vi "AttrGetIsOpen.vi"(5 "LogSuspend":bool, 8 "error in":errorcluster, 11 "UdsHandleIn":T1={"LogPath"=path "", "LogEnabled"=FALSE, "isOpen"=FALSE, "LogContent"="", "Adapter"="CAN0", "MCanHandle"={"MCanAdapter"=refnum}, "TransmittId"=0, "ReceiveId"=0}) -> (0 "error out":errorcluster, 2 "State":bool, 3 "UdsHandleOut":T1={"LogPath"=path "", "LogEnabled"=FALSE, "isOpen"=FALSE, "LogContent"="", "Adapter"="CAN0", "MCanHandle"={"MCanAdapter"=refnum}, "TransmittId"=0, "ReceiveId"=0})   [LabVIEW 2011, in "Konvolucio MUDS150628.lvlib"]
uses:
  <instrlib>/Konvolucio MUDS150628/Konvolucio MUDS150628.lvlib
  <instrlib>/Konvolucio MUDS150628/Types/UdsHandleType.ctl
  <instrlib>/Konvolucio MCAN120803/Types/MCanHandleType.ctl
  C:/Program Files/National Instruments/LabVIEW 2011/instr.lib/Konvolucio MCAN120803/Private/Konvolucio.MCAN120803.dll
  Konvolucio MCAN120803/Private/Konvolucio.MCAN120803.dll
  <instrlib>/Konvolucio MCAN120803/Konvolucio MCAN120803.lvlib
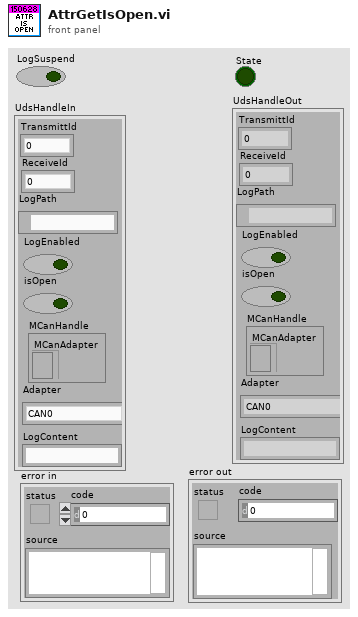
[diagram p1: front panel]
types:
  T1 = typedef "Konvolucio MUDS150628.lvlib/UdsHandleType.ctl" = cluster{"LogPath":path, "LogEnabled":bool, "isOpen":bool, "LogContent":string, "Adapter":string, "MCanHandle":T2, "TransmittId":u32, "ReceiveId":u32}
  T2 = typedef "Konvolucio MCAN120803.lvlib/MCanHandleType.ctl" = cluster{"MCanAdapter":refnum<k24>}
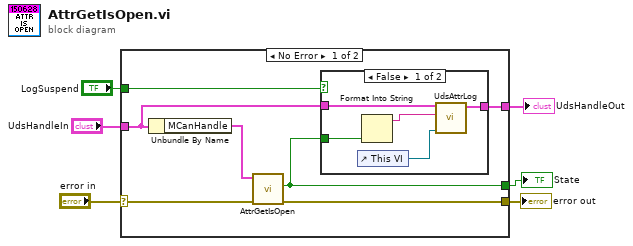
[diagram p0: block diagram]
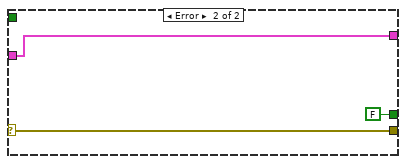
[diagram p3: hidden frame]
diagram:
  n1 = case shown="No Error" "error in" {
    selector: "error in" -> [w9 w22]
    tunnel: [w10 w22] -> w5
    tunnel: "UdsHandleIn" -> [w13 w21]
    tunnel: [w12 w21] -> w2
    tunnel: "LogSuspend" -> [w11 _]
    tunnel: [w7 FALSE ("State")] -> w6
    frame No Error {
      n2 = Unbundle By Name(w13) -> ("MCanHandle"=w8:T2)
      n3 = call <instrlib>:"AttrGetIsOpen.vi"("error in"=w9, "MCanHandleIn"=w8) -> ("error out"=w10:errorcluster, "State"=w7:bool)  [unwired: 7 in, 1 out]
      n4 = case shown="False" w11 {
        tunnel: w13 -> [w18 w19]
        tunnel: [w17 w19] -> w12
        tunnel: w7 -> [w15 _]
        frame False {
          n5 = control-ref of="This VI"() -> (w16:refnum<vi>)
          n6 = Format Into String(w15) -> (resulting string=w14:string)  [unwired: 3 in, 1 out]
          n7 = call <instrlib>:"UdsAttrLog.vi"("This VI"=w16, "Content"=w14, "UdsHandleIn"=w18) -> ("UdsHandleOut"=w17:T1)  [unwired: 8 in]
        }
        frame True {
        }
      }
    }
    frame Error {
    }
  }
  "State" <- w6
  "error out" <- w5
  "UdsHandleOut" <- w2
